vi "Generate Offset Histogram.vi"(11 "Data In":dbl[](array[numeric])) -> ()   [LabVIEW 2014, in "Analysis.lvlib"]
uses:
  Analysis.lvlib
  <vilib>/Analysis/NI_AALBase.lvlib
panel:
  out "Histogram Graph":T1(graph)
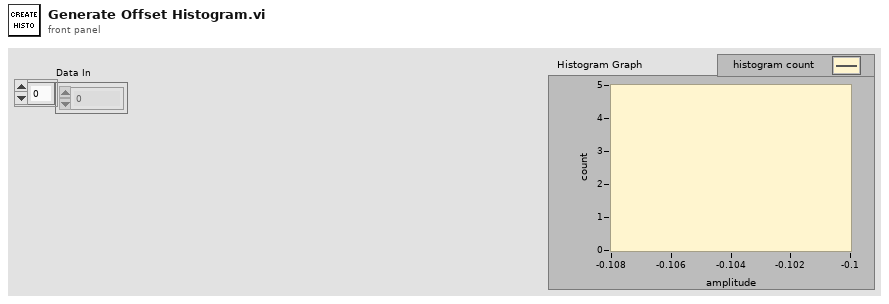
[diagram p1: front panel]
types:
  T1 = cluster{"X Values":dbl[], "Histogram: h(x)":i32[]}
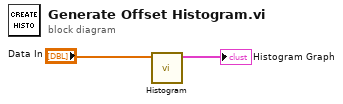
[diagram p0: block diagram]
diagram:
  n1 = call <vilib>:"Histogram.vi"("X"="Data In") -> ("Histogram Graph"=→"Histogram Graph":T1)  [unwired: 7 in, 3 out]
